vi "SelectROI.vi"(8 "error in (no error)":errorcluster, 11 "Image in":T1) -> (0 "error out":errorcluster, 1 "Global Rectangle Roy":i32[](array[numeric]), 2 "Global Rectangle Rob":i32[](array[numeric]), 3 "Image out":T1)   [LabVIEW 2012]
uses:
  <vilib>/vision/Image Controls.llb/IMAQ Image.ctl
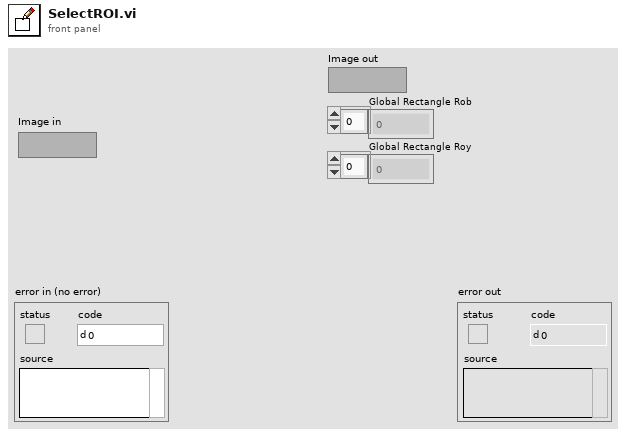
[diagram p1: front panel]
types:
  T1 = typedef "IMAQ Image.ctl" = refnum<image>
  T2 = typedef "ROI Descriptor" = cluster{"Global Rectangle":i32[], "Contours":cluster{"ID":enum32{"External", "Internal"}, "Type":u32, "Coordinates":i32[]}[]}
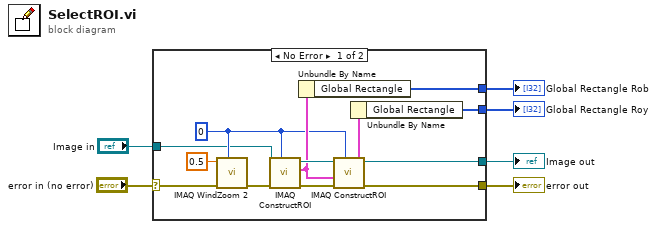
[diagram p0: block diagram]
diagram:
  n1 = case shown="No Error" "error in (no error)" {
    selector: "error in (no error)" -> [w15 w21]
    tunnel: [w12 w21] -> w5
    tunnel: "Image in" -> [w10 w20]
    tunnel: [w9 w20] -> w3
    tunnel: [w8 _] -> w2
    tunnel: [w7 _] -> w1
    frame No Error {
      w13 = 0 ("Window Number (0...15)")
      n2 = call "IMAQ WindZoom 2"("Window Number (0...15)"=w13, "error in (no error)"=w15, "Zoom Factor"=sgl 0.5) -> ("error out"=w14:errorcluster)  [unwired: 5 in, 3 out]
      n3 = call "IMAQ ConstructROI"("Window Number (-1...15)"=w13, "error in (no error)"=w14, "Image"=w10) -> ("error out"=w18:errorcluster, "ROI Descriptor Out"=w17:T2, "Image Out (duplicate)"=w19:T1)  [unwired: 5 in, 1 out]
      n4 = Unbundle By Name(w17) -> ("Global Rectangle"=w8:i32[])
      n5 = call "IMAQ ConstructROI"("Window Number (-1...15)"=w13, "error in (no error)"=w18, "ROI Descriptor In (None)"=w17, "Image"=w19) -> ("error out"=w12:errorcluster, "ROI Descriptor Out"=w16:T2, "Image Out (duplicate)"=w9:T1)  [unwired: 4 in, 1 out]
      n6 = Unbundle By Name(w16) -> ("Global Rectangle"=w7:i32[])
    }
    frame Error {
    }
  }
  "error out" <- w5
  "Image out" <- w3
  "Global Rectangle Rob" <- w2
  "Global Rectangle Roy" <- w1
